vi "RCL Waveform State.vi"(8 "error in (no error)":errorcluster, 11 "Actor_Scope in":refnum<class "Actor_Scope.lvclass">) -> (0 "error out":errorcluster, 3 "Actor_Scope out":refnum<class "Actor_Scope.lvclass">)   [LabVIEW 2020, in "Actor_Scope.lvlib" / "Actor_Scope.lvclass"]
uses:
  Actor_Scope.lvclass
  Actor_Scope.lvclass/Actor_Scope.ctl
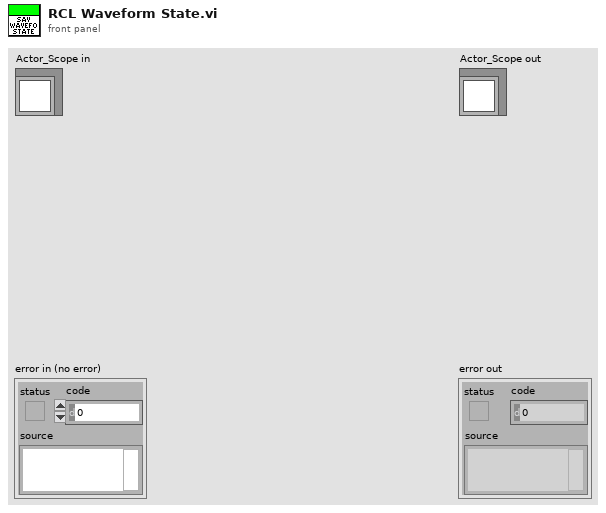
[diagram p1: front panel]
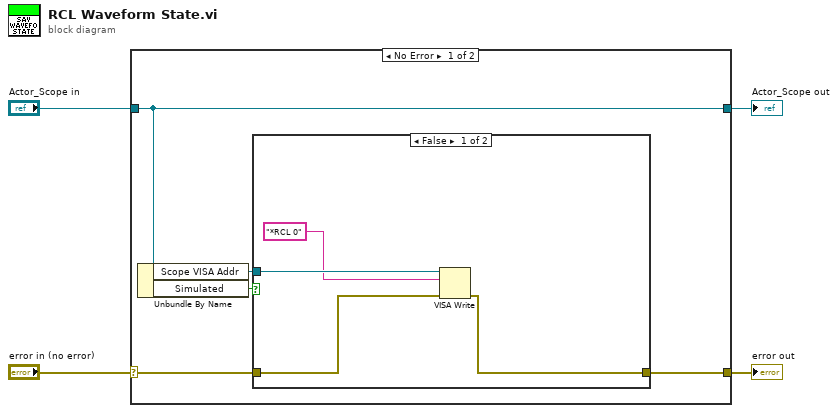
[diagram p0: block diagram]
diagram:
  n1 = case shown="No Error" "error in (no error)" {
    selector: "error in (no error)" -> [w7 w16]
    tunnel: [w6 w16] -> w3
    tunnel: [w9 w15] -> w1
    tunnel: "Actor_Scope in" -> [w9 w15]
    frame No Error {
      n2 = Unbundle By Name(w9) -> ("Scope VISA Addr"=w5:refnum<visa-resource-name>, "Simulated"=w8:bool)
      n3 = case shown="False" w8 {
        tunnel: w7 -> [w11 w14]
        tunnel: [w10 w14] -> w6
        tunnel: w5 -> [w13 _]
        frame False {
          n4 = VISA Write(VISA resource name=w13, write buffer="*RCL 0", error in (no error)=w11) -> (error out=w10:errorcluster)  [unwired: 2 out]
        }
        frame True {
        }
      }
    }
    frame Error {
    }
  }
  "error out" <- w3
  "Actor_Scope out" <- w1
